vi "PipBoy_EnqueueIfDontExist.vi"(8 "error in (no error)":errorcluster, 9 "Message Data":variant, 10 "Message":string="AcquirePipBoy", 11 "Message Queue":refnum<queue>) -> (0 "error out":errorcluster)   [LabVIEW 2014]
uses:
  modules/support/Message Queue/Message Cluster.ctl
  modules/support/Message Queue/Message Queue.lvlib
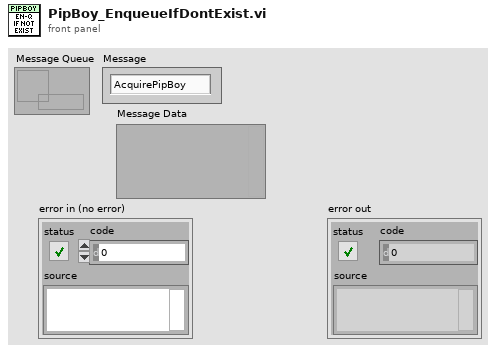
[diagram p1: front panel]
types:
  T1 = typedef "Message Queue.lvlib/Message Cluster.ctl" = cluster{"Message":string, "Message Data":variant}
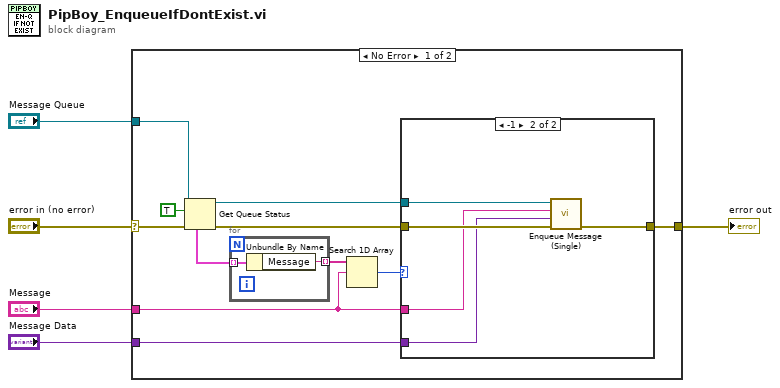
[diagram p0: block diagram]
diagram:
  n1 = case shown="No Error" "error in (no error)" {
    selector: "error in (no error)" -> [w13 w25]
    tunnel: "Message Queue" -> [w12 _]
    tunnel: [w14 w25] -> w4
    tunnel: "Message" -> [w7 _]
    tunnel: "Message Data" -> [w11 _]
    frame No Error {
      n2 = Get Queue Status(queue=w12, return elements? (F)=TRUE, error in (no error)=w13) -> (queue out=w15:refnum<queue>, error out=w16:errorcluster, elements=w9:T1[])  [unwired: 5 out]
      n3 = for {
        tunnel: w9 -> [w18] mode=indexing
        tunnel: [w17] -> w8 mode=indexing
        n4 = Unbundle By Name(w18) -> ("Message"=w17:string)
      }
      n5 = Search 1D Array(1D array=w8, element=w7) -> (index of element=w6:i32)  [unwired: 1 in]
      n6 = case shown="-1" w6 {
        tunnel: w16 -> [w19 w24]
        tunnel: w15 -> [_ w23]
        tunnel: [w19 w22] -> w14
        tunnel: w7 -> [_ w21]
        tunnel: w11 -> [_ w20]
        frame Default {
        }
        frame -1 {
          n7 = call "Enqueue Message (Single).vi"("error in (no error)"=w24, "Message Data"=w20, "Message"=w21, "Message Queue"=w23) -> ("error out"=w22:errorcluster)  [unwired: 6 in, 1 out]
        }
      }
    }
    frame Error {
    }
  }
  "error out" <- w4
